vi "GetDependentTypeDefs.vi"(8 "error in (no error)":errorcluster, 10 "vi name":string, 11 "app reference in":refnum<vi>) -> (0 "error out":errorcluster, 2 "Dependendent TypeDefs wParents":T1[](array[typedef]), 3 "app reference out":refnum<vi>)   [LabVIEW 2013, in "DiscoverCommonTypeDefCallers.lvlib"]
doc: "Takes a single VI name (as a string) as input and finds all TypeDefs that the specified VI is dependent upon -- that is, directly uses. SubVIs called by the specified VI are NOT searched for their dependent TypeDefs. The output is an array of TypeDef names (as strings)."
uses:
  DiscoverCommonTypeDefCallers.lvlib
  DependendentTypeDefwParents.ctl
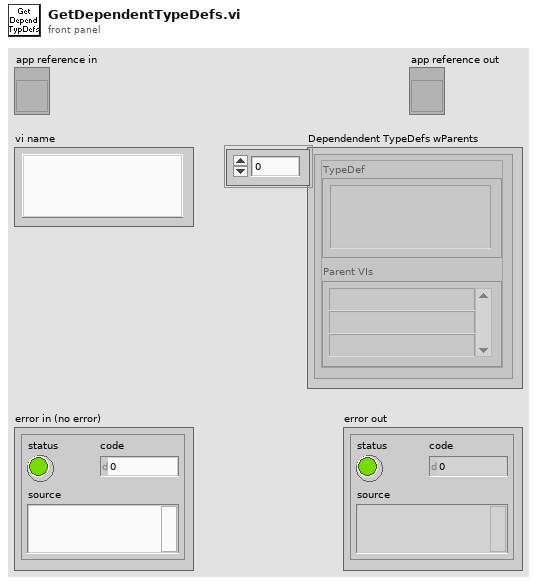
[diagram p1: front panel]
types:
  T1 = typedef "DiscoverCommonTypeDefCallers.lvlib/DependendentTypeDefwParents.ctl" = cluster{"TypeDef":string, "Parent VIs":string[]}
  T2 = enum32{"not a control VI", "control", "typedef", "strict typedef"}
  T3 = enum32{"invalid VI type", "Standard VI", "Control VI", "Global VI", "Polymorphic VI", "Configuration VI", "SubSystem", "Facade VI", "Method VI", "Statechart Diagram VI"}
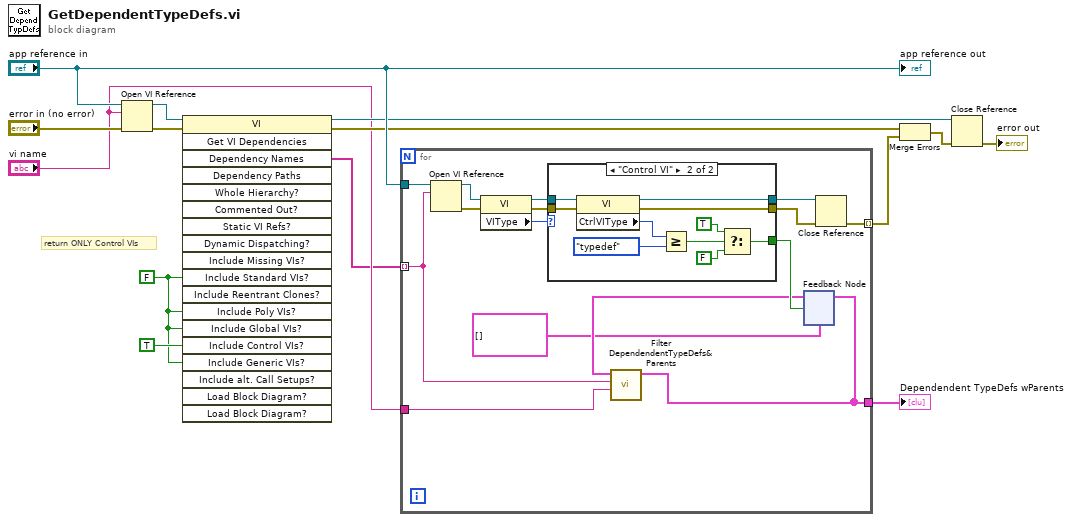
[diagram p0: block diagram]
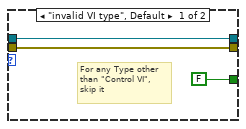
[diagram p2: hidden frame]
diagram:
  w10 = FALSE ("Include Global VIs?")
  # "return ONLY Control VIs"
  n1 = Open VI Reference(application reference (local)="app reference in", vi path="vi name", error in (no error)="error in (no error)") -> (vi reference=w14:refnum<vi>, error out=w12:errorcluster)  [unwired: 3 in]
  n2 = invoke class="VI" method="Get VI Dependencies"(reference=w14, error in=w12, "Include Standard VIs?"=w10, "Include Poly VIs?"=w10, "Include Global VIs?"=w10, "Include Control VIs?"=TRUE, "Include Generic VIs?"=w10) -> (reference out=w8:refnum<vi>, error out=w7:errorcluster, "Dependency Names"=w2:string[])  [unwired: 12 in, 16 out]
  n3 = for {
    tunnel: w2 -> [w19] mode=indexing
    tunnel: "app reference in" -> [w25]
    tunnel: [w21] -> w4 mode=indexing
    tunnel: "vi name" -> [w17]
    tunnel: [w15] -> w1
    n4 = Open VI Reference(application reference (local)=w25, vi path=w19) -> (vi reference=w24:refnum<vi>, error out=w26:errorcluster)  [unwired: 4 in]
    n5 = property class="VI"(reference=w24, error in=w26) -> (reference out=w29:refnum<vi>, error out=w28:errorcluster, "VIType"=w27:T3)
    n6 = case shown="\"Control VI\"" w27 {
      tunnel: w29 -> [w32 w42]
      tunnel: w28 -> [w31 w41]
      tunnel: [w31 w40] -> w22
      tunnel: [w32 w39] -> w23
      tunnel: [FALSE w33] -> w20
      frame "invalid VI type", Default {
        # "For any Type other \nthan \"Control VI\", skip it"
      }
      frame "Control VI" {
        n7 = property class="VI"(reference=w42, error in=w41) -> (reference out=w39:refnum<vi>, error out=w40:errorcluster, "CtrlVIType"=w37:T2)
        n8 = Greater Or Equal?(x=w37, y=T2."typedef" ("Control VI Type")) -> (x >= y?=w34:bool)
        n9 = Select(t=TRUE, s=w34, f=FALSE) -> (s? t:f=w33:bool)
      }
    }
    n10 = feedback #1(T1[] [] ("Dependendent TypeDefs wParents (out)")) -> (w18:T1[])
    n11 = call "Filter DependendentTypeDefs&Parents.vi"("Parent VI Name"=w17, "Dependency Name"=w19, "Dependendent TypeDefs wParents (in)"=w18) -> ("Dependendent TypeDefs wParents (out)"=w15:T1[])  [unwired: 8 in]
    n12 = feedback-in #1(w15, w20) -> ()
    n13 = Close Reference(reference=w23, error in (no error)=w22) -> (error out=w21:errorcluster)
  }
  "Dependendent TypeDefs wParents" <- w1
  n14 = Merge Errors(w7, w4) -> (w5:errorcluster)
  n15 = Close Reference(reference=w8, error in (no error)=w5) -> (error out=→"error out":errorcluster)
  "app reference out" <- "app reference in"
